vi "Visualizacion_NEW.vi"() -> ()   [LabVIEW 2021]
uses:
  <vilib>/Modbus/master/Modbus Master.lvclass
  4cb8985d-a683-42ab-be0b-9e8f42a2c2d0.vi
  <vilib>/Analysis/NI_AALBase.lvlib
  <vilib>/Modbus/master/Create Master Instance (TCP).vi
  <vilib>/Analysis/baseanly.llb/Mean (DBL).vi
panel:
  in  "Save Parameters":bool
  in  "Activar sim Bitron":bool
  out "MEDIA TEMPERATURAS":dbl format="%0.2f"
  out "Peltiers enable":bool
  out "Program Status":bool
  out "SP (T)":sgl
  out "Segmento_temp":u16
  in  "?":T1(tab)
  out "Temp Valve 1":sgl format="%#.2g"
  out "Temp Bobina 1":sgl
  out "PWM 1(SP)":u16
  out "PWM 2(SP)":u16
  out "Temp Valve 2":sgl format="%#.2g"
  out "Temp Bobina 2":sgl
  out "PWM 3(SP)":u16
  out "Temp Bobina 3":sgl
  out "Temp Valve 3":sgl format="%#.2g"
  out "PWM 4(SP)":u16
  out "Temp Valve 4":sgl format="%#.2g"
  out "Temp Bobina 4":sgl
  out "Temp Valve 5":sgl
  out "Temp Bobina 5":sgl
  out "PWM 5(SP)":u16
  out "PWM 6(SP)":u16
  out "Temp Valve 6":sgl format="%#.2g"
  out "Temp Bobina 6":sgl
  out "PWM 7(SP)":u16
  out "Temp Valve 7":sgl format="%#.2g"
  out "Temp Bobina 7":sgl
  out "PWM 8":u16
  out "Temp Bobina 8":sgl
  out "Temp Valve 8":sgl format="%#.2g"
  in  "?":T2(tab)
  in  "?":T3(tab)
  out "TEMPERATURA MEDIA":dynamicdata(graph)
  out "ALL TOGETHER":dynamicdata(graph)
  out "VALVULA 1 Y BOBINA 1":dynamicdata(graph)
  out "VALVULA 2 Y BOBINA 2":dynamicdata(graph)
  out "VALVULA 3 Y BOBINA 3":dynamicdata(graph)
  out "VALVULA 4 Y BOBINA 4":dynamicdata(graph)
  out "VALVULA 5  Y BOBINA 5":dynamicdata(graph)
  out "VALVULA 6 Y BOBINA 6":dynamicdata(graph)
  out "VALVULA 7 Y BOBINA 7":dynamicdata(graph)
  out "VALVULA 8 Y PELTIER 8":dynamicdata(graph)
  out "Camara climatica":dynamicdata(graph)
  out "W1.16":bool
  out "W1.15":bool
  out "W1.11":bool
  out "1.10":bool
  out "W1.14":bool
  out "W1.13":bool
  out "W1.12":bool
  out "W1.1":bool
  out "W2":bool
  out "W3":bool
  out "W4":bool
  out "W1.2":bool
  out "W1.3":bool
  out "W1.6":bool
  out "W1.5":bool
  out "W1.4":bool
  out "W1.9":bool
  out "W1.8":bool
  out "W1.7":bool
  out "warnings table":T4(array[cluster]) {"Time Stamp" format="%<%.3X %x>T"}
  in  "Reset":bool
  in  "Pelt ºC/min":dbl=2.5
  in  "Cam ºC/min":dbl=2.2
  in  "Tiempo máximo de ciclo(min)":dbl=90.0
  in  "Setpoint corte frío(ºC)":dbl=-30.0
  in  "Setpoint Frío(ºC)":dbl=-40.0
  in  "Setpoint peltiers(ºC)":dbl=85.0
  in  "Tiempo estabilidad de Frío(min)":dbl=15.0
  in  "Tiempo mínimo de ciclo(min)":dbl=70.0
  in  "Setpoint calor corte rampa(ºC)":dbl=51.0
  in  "T ciclo (Bitron FSM Sim)":dbl=90.0
  in  "Setpoint calor cam":dbl=55.0
  out "DO H2 Lab":bool
  in  "Guardar datos":bool=TRUE
  out "Array":dbl[][](array[numeric])
  out "Guardando en disco":bool
  out "array w/ subset deleted":dbl[][](array[numeric])
  out "Guardar Array":dbl[][](array[numeric])
  out "size(s)":i32
  out "senal_bitron":bool
  in  "Stop Control Program":bool
  out "Coils write":bool[](array[boolean])
  out "error out":errorcluster
  out "Int values":u16[](array[numeric])
  out "SGL values":sgl[](array[numeric])
  out "coil values":bool[](array[boolean])
  out "ComunicacionCRIO":bool
  out "current time":timestamp
  in  "run_program":bool
  out "Setpoint_temp_write":dbl
  out "Setpoint_hum_write":dbl
  out "Setpoint_temp_read":dbl
  out "Setpoint_hum_read":dbl
  in  "Pause_Entrar_camara":bool
  in  "Pause":bool
  in  "stop":bool
  # "Control Programa Principal"
  # "Cámara climática"
  # "ºC"
  # "ºC"
  # "%"
  # "%"
  # "Simulación señal Bitron"
  # "ºC"
  # "Peltier 1"
  # "ºC"
  # "ºC"
  # "Peltier 2"
  # "ºC"
  # "ºC"
  # "Peltier 3"
  # "ºC"
  # "ºC"
  # "Peltier 4"
  # "ºC"
  # "Peltier 5 (Doble)"
  # "ºC"
  # "ºC"
  # "Peltier 6 (Doble)"
  # "ºC"
  # "ºC"
  # "Peltier 7 (Doble)"
  # "ºC"
  # "ºC"
  # "Peltier 8 (Doble)"
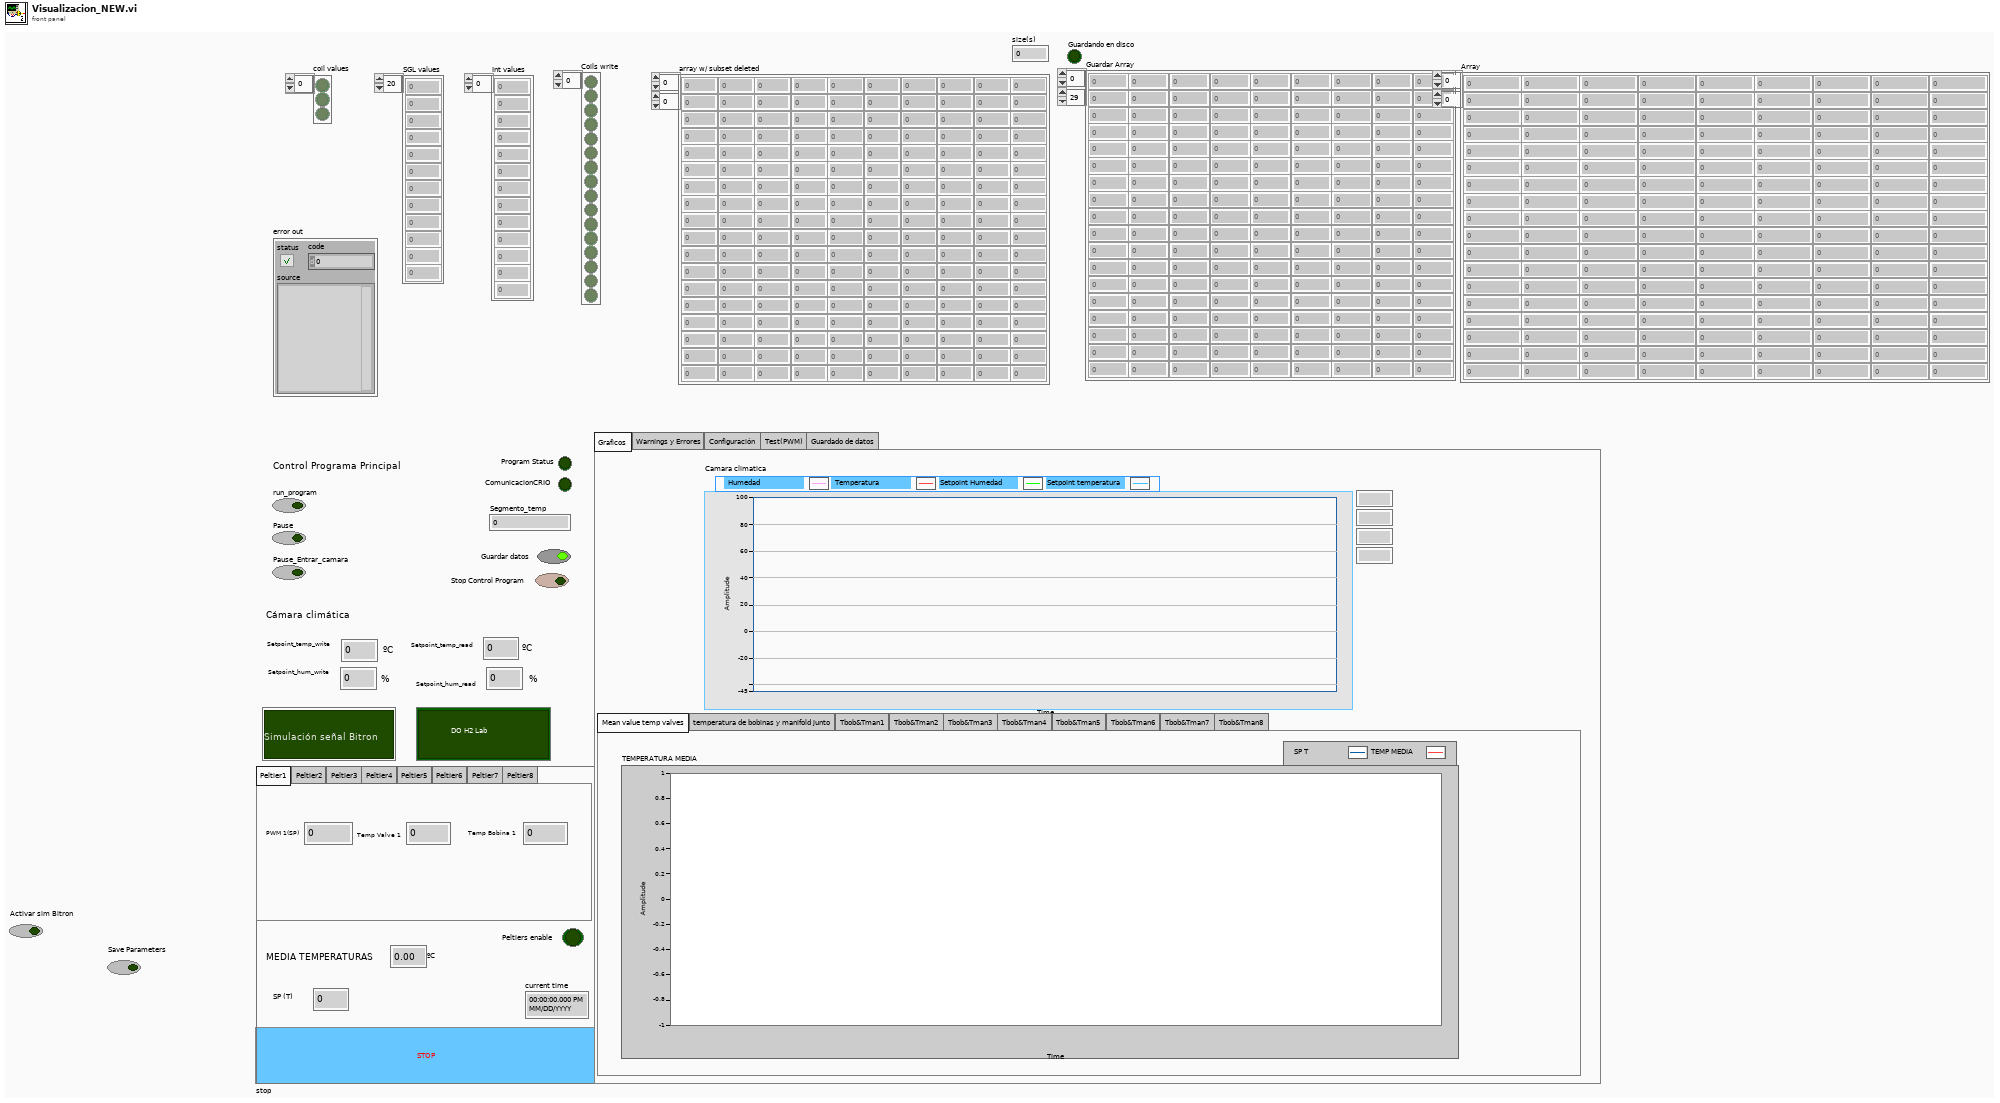
[diagram p1: front panel]
types:
  T1 = enum32{"Peltier1", "Peltier2", "Peltier3", "Peltier4", "Peltier5", "Peltier6", "Peltier7", "Peltier8"}
  T2 = enum32{"Graficos", "Warnings y Errores", "Configuración", "Test(PWM)", "Guardado de datos"}
  T3 = enum32{"Mean value temp valves", "temperatura de bobinas y manifold junto", "Tbob&Tman1", "Tbob&Tman2", "Tbob&Tman3", "Tbob&Tman4", "Tbob&Tman5", "Tbob&Tman6", "Tbob&Tman7", "Tbob&Tman8"}
  T4 = cluster{"Time Stamp":timestamp, "Descripcion":string, "Numeric":i32}[]
  T5 = enum16{"open", "open or create", "create or replace", "create", "open (read-only)"}
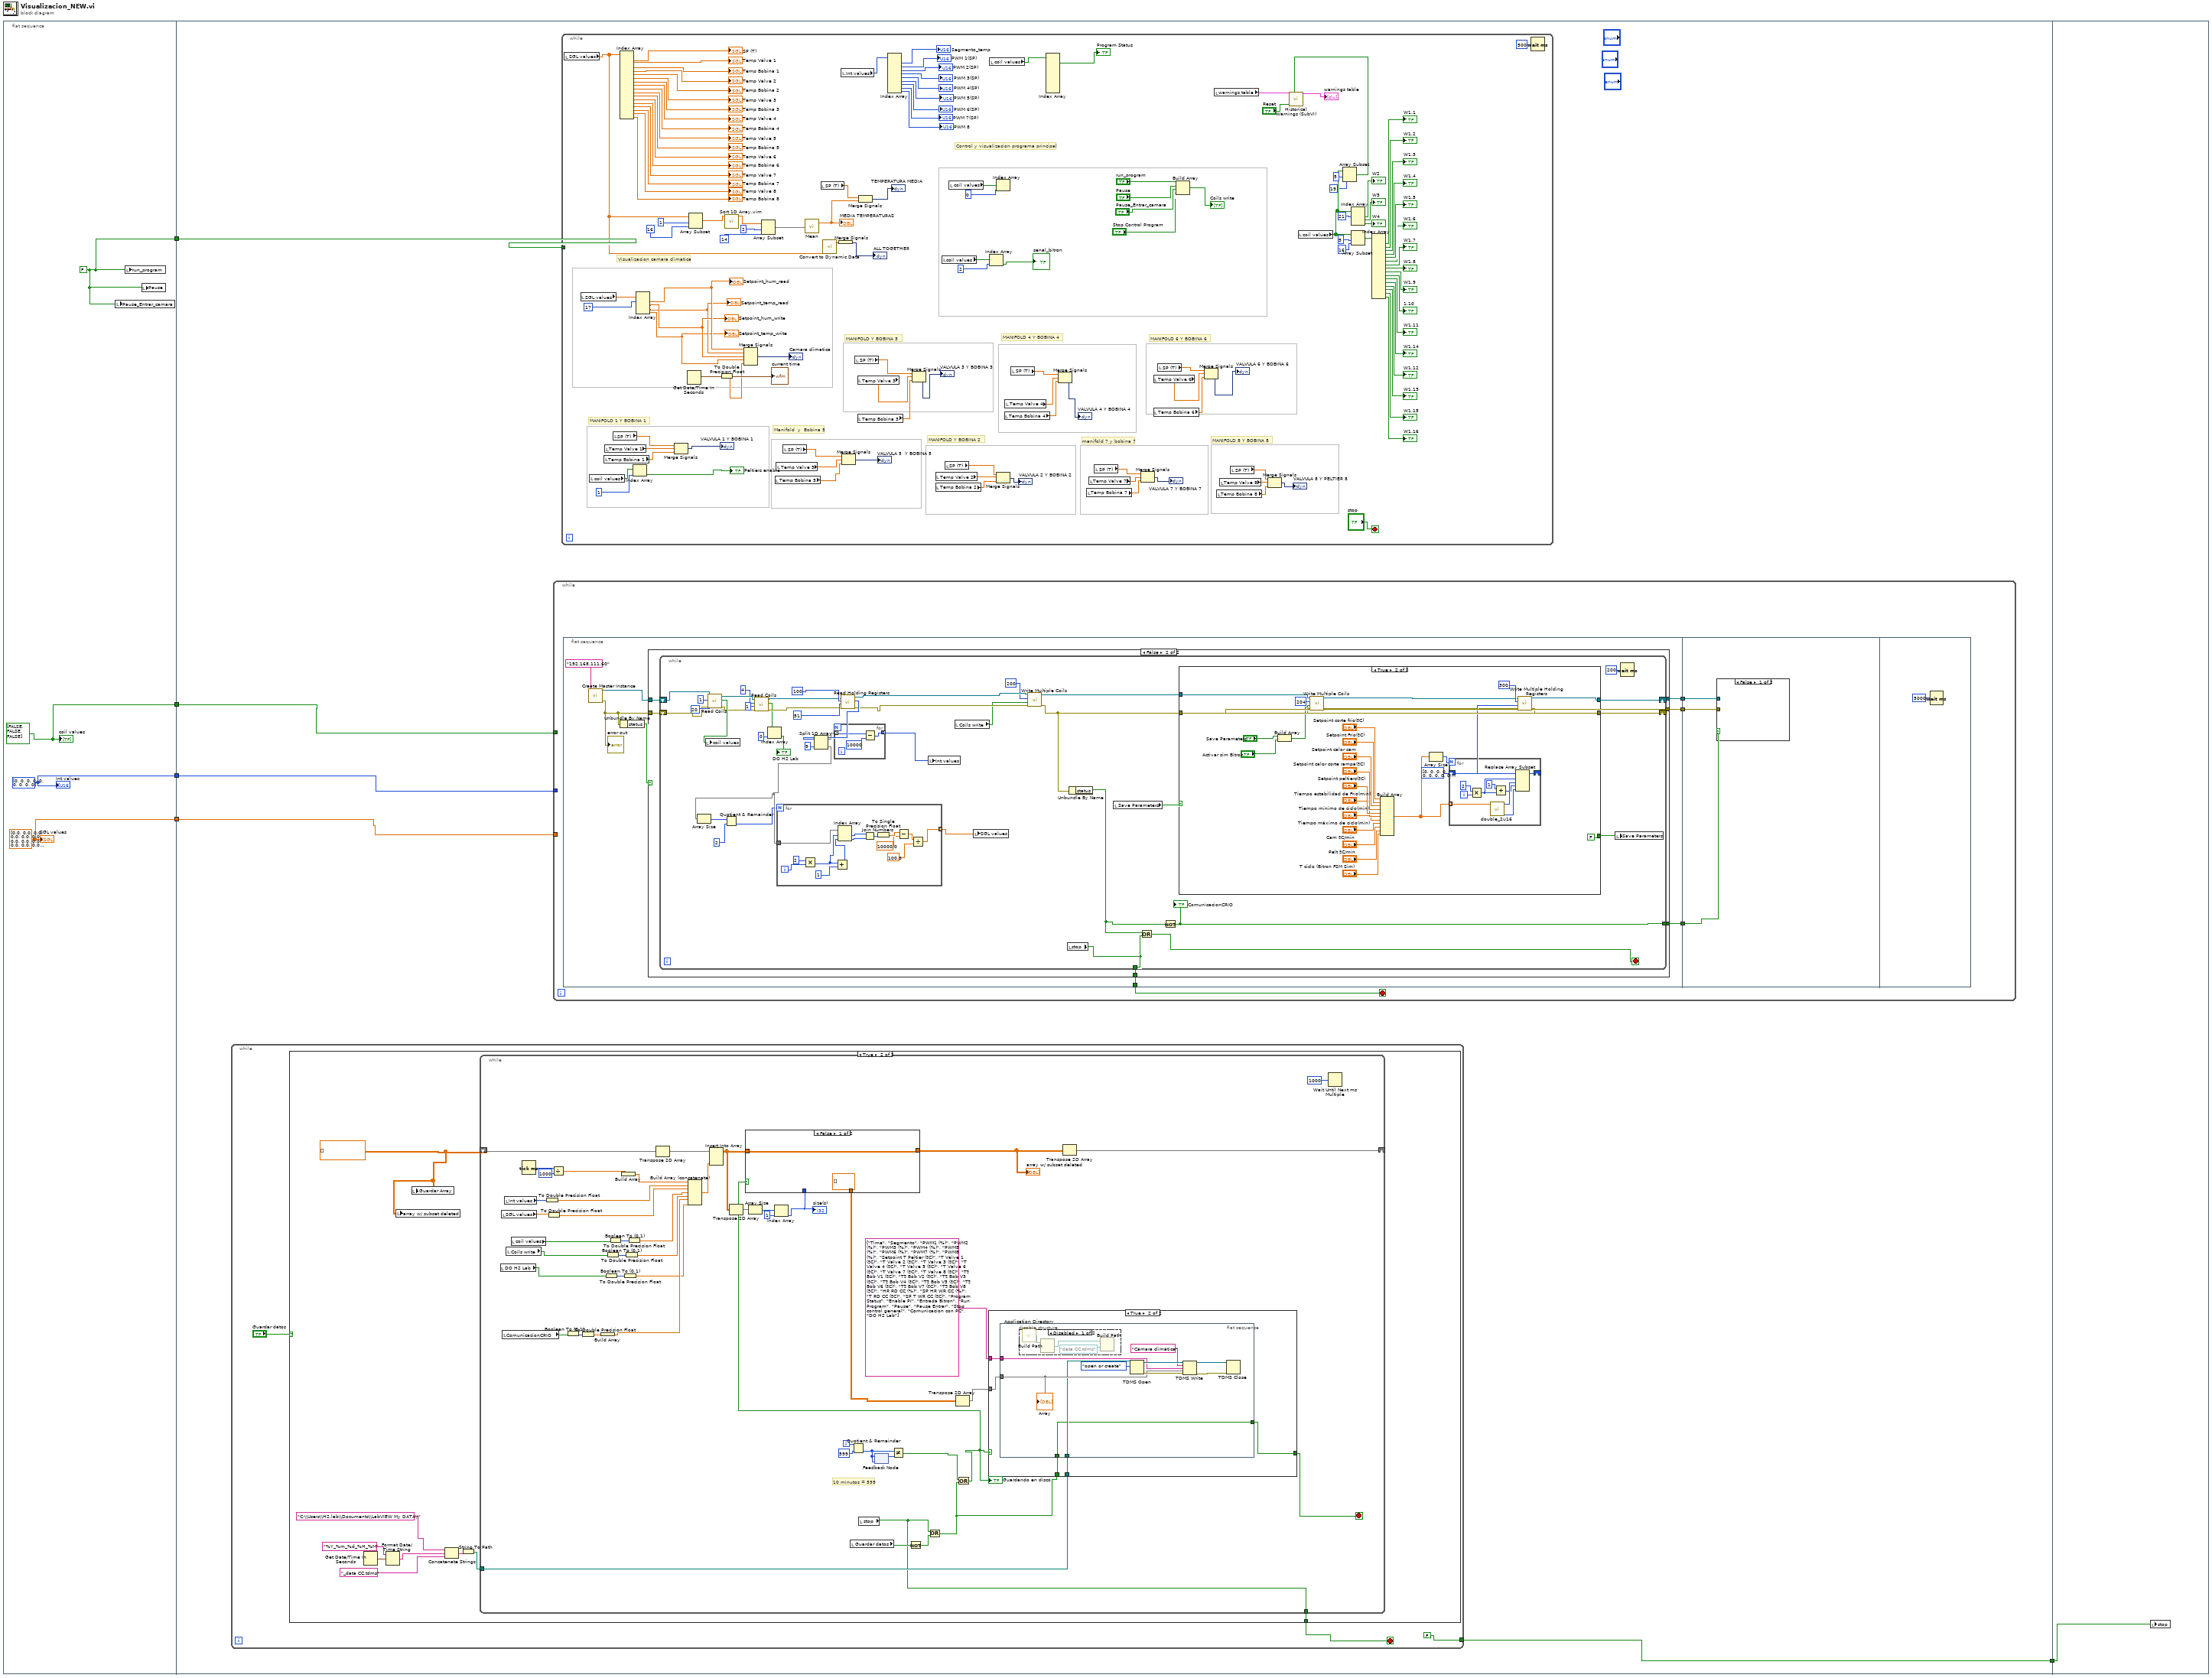
[diagram p0: block diagram]
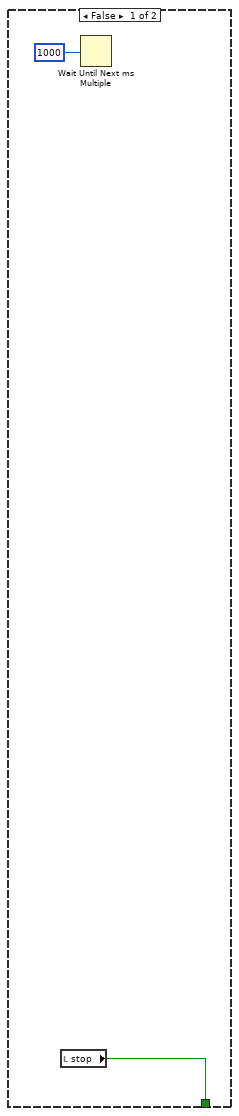
[diagram p2: hidden frame]
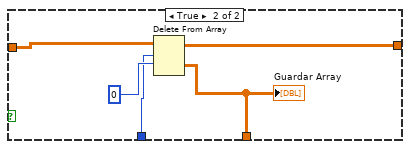
[diagram p3: hidden frame]
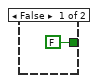
[diagram p4: hidden frame]
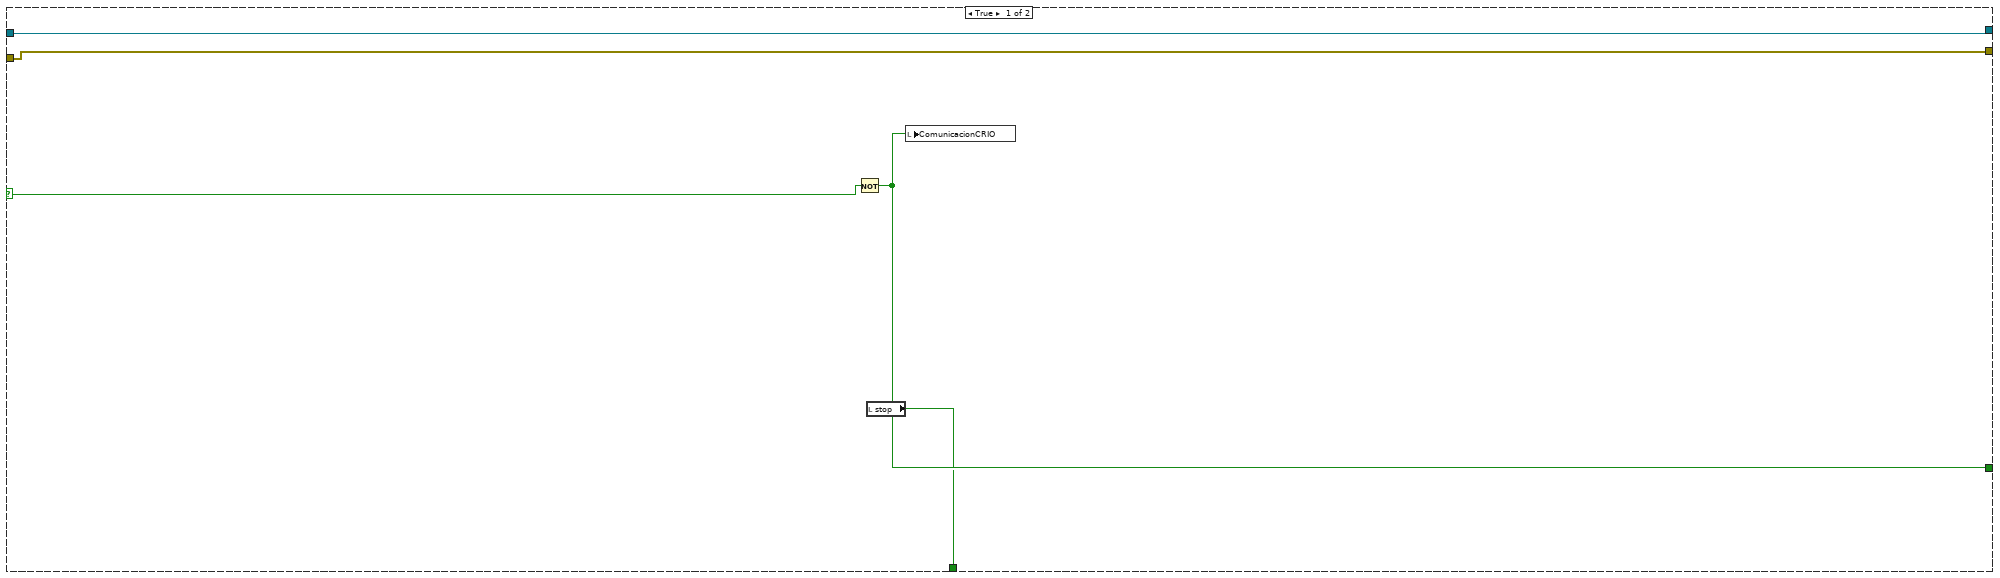
[diagram p6: hidden frame]
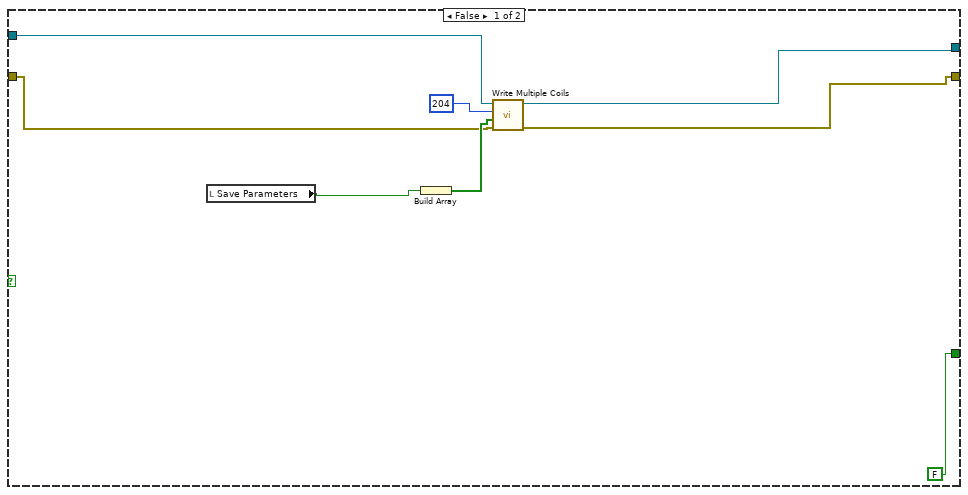
[diagram p7: hidden frame]
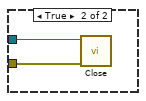
[diagram p8: hidden frame]
diagram:
  n1 = flat-sequence {
    tunnel: [w9] -> w5
    tunnel: [w8] -> w4
    tunnel: [w7] -> w3
    tunnel: [w6] -> w2
    tunnel: w5 -> [w14]
    tunnel: w4 -> [w13]
    tunnel: w3 -> [w12]
    tunnel: w2 -> [w11]
    tunnel: [w10] -> w1
    tunnel: w1 -> [w361]
    frame #0 {
      w7 = sgl[] [0.0, 0.0, 0.0, 0.0, 0.0, 0.0, 0.0, 0.0, 0.0, 0.0, 0.0, 0.0, 0.0, 0.0, 0.0, 0.0, 0.0, 0.0, 0.0, 0.0, 0.0] ("SGL values")
      w8 = u16[] [0, 0, 0, 0, 0, 0, 0, 0, 0] ("Int values")
      w6 = FALSE ("run_program")
      w9 = bool[] [FALSE, FALSE, FALSE] ("coil values")
      n2 = local write "Pause_Entrar_camara"(w6) -> ()
      n3 = local write "run_program"(w6) -> ()
      n4 = local write "Pause"(w6) -> ()
      "coil values" <- w9
      "Int values" <- w8
      "SGL values" <- w7
    }
    frame #1 {
      n5 = while {
        tunnel: [FALSE ("stop Control General")] -> w10
        stop <- w16 stop-if-true
        n6 = case shown="True" "Guardar datos" {
          tunnel: [w18 w20] -> w16
          frame False {
            n7 = local read "stop"() -> (w18:bool)
            n8 = Wait Until Next ms Multiple(millisecond multiple=u32 1000 ("milliseconds to wait")) -> ()  [unwired: 1 out]
          }
          frame True {
            w28 = dbl[][] []
            n9 = Get Date/Time In Seconds() -> (seconds since 1Jan1904=w27:timestamp)
            n10 = Format Date/Time String(time format string (%c)="%Y_%m_%d_%H_%M", seconds (now)=w27) -> (date/time string=w24:string)  [unwired: 1 in]
            n11 = local write "array w/ subset deleted"(w28) -> ()
            n12 = local write "Guardar Array"(w28) -> ()
            n13 = Concatenate Strings("C:\\Users\\H2.lab\\Documents\\LabVIEW My DATA\\" ("string"), w24, "_data CC.tdms" ("string")) -> (w25:string)
            n14 = String To Path(string=w25) -> (path=w22:path)
            n15 = while {
              shift-right: [w65] -> _
              shift-left: w28 -> [w68]
              tunnel: w22 -> [w56]
              tunnel: [w32] -> w20
              i -> [w73]
              stop <- w36 stop-if-true
              # "10 minutos = 599"
              n16 = local read "DO H2 Lab"() -> (w30:bool)
              n17 = local read "SGL values"() -> (w54:sgl[])
              n18 = local read "ComunicacionCRIO"() -> (w38:bool)
              n19 = local read "Int values"() -> (w55:u16[])
              n20 = local read "Coils write"() -> (w40:bool[])
              n21 = local read "coil values"() -> (w43:bool[])
              n22 = Tick Count (ms)() -> (millisecond timer value=w59:u32)
              n23 = To Double Precision Float(number=w55) -> (double precision float=w53:dbl[])
              n24 = To Double Precision Float(number=w54) -> (double precision float=w52:dbl[])
              n25 = Divide(x=w59, y=u32 1000) -> (x/y=w51:dbl)
              n26 = Boolean To (0,1)(Boolean=w38) -> (0, 1=w47:i16)
              n27 = To Double Precision Float(number=w47) -> (double precision float=w46:dbl)
              n28 = Build Array(w46) -> (w42:dbl[])
              n29 = Boolean To (0,1)(Boolean=w30) -> (0, 1=w31:i16)
              n30 = Boolean To (0,1)(Boolean=w40) -> (0, 1=w41:i16[])
              n31 = Boolean To (0,1)(Boolean=w43) -> (0, 1=w49:i16[])
              n32 = Build Array(w51) -> (w50:dbl[])
              n33 = To Double Precision Float(number=w31) -> (double precision float=w29:dbl)
              n34 = To Double Precision Float(number=w41) -> (double precision float=w39:dbl[])
              n35 = To Double Precision Float(number=w49) -> (double precision float=w48:dbl[])
              n36 = Transpose 2D Array(2D array=w68) -> (transposed array=w67:dbl[][])
              n37 = Build Array (concatenate)(w50, w53, w52, w48, w39, w42, w29) -> (w74:dbl[])
              n38 = Insert Into Array(array=w67, new element=w74) -> (w70:dbl[][])  [unwired: 2 in]
              n39 = Transpose 2D Array(2D array=w70) -> (transposed array=w64:dbl[][])
              n40 = Array Size(array=w64) -> (size(s)=w63:i32[])
              n41 = Index Array(array=w63, index=1) -> (element=w62:i32)
              "size(s)" <- w62
              n42 = local read "Guardar datos"() -> (w35:bool)
              n43 = Quotient & Remainder(x=w73, y=599) -> (floor(x/y)=w69:i32)  [unwired: 1 out]
              n44 = local read "stop"() -> (w32:bool)
              n45 = feedback-in #1(w69) -> ()
              n46 = feedback #1(w69) -> (w71:i32)
              n47 = Not Equal?(x=w69, y=w71) -> (x != y?=w37:bool)
              n48 = Not(x=w35) -> (.not. x?=w34:bool)
              n49 = Or(x=w32, y=w34) -> (x .or. y?=w33:bool)
              n50 = Or(x=w37, y=w33) -> (x .or. y?=w45:bool)
              "Guardando en disco" <- w45
              n51 = case shown="False" w45 {
                tunnel: w70 -> [w77 w80]
                tunnel: [w77 w82] -> w66
                tunnel: w62 -> [_ w79]
                tunnel: [dbl[][] [] w78] -> w44
                frame False {
                }
                frame True {
                  n52 = Delete From Array(array=w80, length=w79, index (row)=0) -> (deleted portion=w78:dbl[][], array with subset deleted=w82:dbl[][])  [unwired: 1 in]
                  "Guardar Array" <- w78
                }
              }
              "array w/ subset deleted" <- w66
              n53 = Transpose 2D Array(2D array=w44) -> (transposed array=w60:dbl[][])
              n54 = case shown="True" w45 {
                tunnel: string[] ["Time", "Segmento", "PWM1 (%)", "PWM2 (%)", "PWM3 (%)", "PWM4 (%)", "PWM5 (%)", "PWM6 (%)", "PWM7 (%)", "PWM8 (%)", "Setpoint T Peltier (ºC)", "T Valve 1 (ºC)", "T Valve 2 (ºC)", "T Valve 3 (ºC)", "T Valve 4 (ºC)", "T Valve 5 (ºC)", "T Valve 6 (ºC)", "T Valve 7 (ºC)", "T Valve 8 (ºC)", "Tª Bob V1 (ºC)", "Tª Bob V2 (ºC)", "Tª Bob V3 (ºC)", "Tª Bob V4 (ºC)", "Tª Bob V5 (ºC)", "Tª Bob V6 (ºC)", "Tª Bob V7 (ºC)", "Tª Bob V8 (ºC)", "HR RD CC (%)", "SP HR WR CC (%)", "T RD CC (ºC)", "SP T WR CC (ºC)", "Program Status", "Enable PI", "Entrada Bitron", "Run Program", "Pause", "Pause Entrar", "Stop control general", "Comunicacion con PC", "DO H2 Lab"] -> [_ w88]
                tunnel: w60 -> [_ w87]
                tunnel: w56 -> [_ w86]
                tunnel: w33 -> [_ w85]
                tunnel: [FALSE ("STOP ALL") w84] -> w36
                frame False {
                }
                frame True {
                  n55 = flat-sequence {
                    tunnel: w88 -> [w94]
                    tunnel: w87 -> [w91]
                    tunnel: w86 -> [w90]
                    tunnel: w85 -> [w89]
                    tunnel: [w89] -> w84
                    frame #0 {
                      n56 = disable-structure shown="Disabled" {
                        frame Disabled {
                          n57 = call <vilib>:"Application Directory.vi"() -> ("Application Directory"=w100:path)
                          n58 = Build Path(base path=w100) -> (appended path=w99:path)  [unwired: 1 in]
                          n59 = Build Path(base path=w99, name or relative path=path "data CC.tdms") -> ()  [unwired: 1 out]
                        }
                        frame Enabled {
                        }
                      }
                      n60 = TDMS Open(10:T5."open or create" ("operation (0:open)"), 11:w90) -> (0:w96:errorcluster, 3:w97:refnum<k34>)  [unwired: 5 in]
                      n61 = TDMS Write(0:w97, 5:"Cámara climática" ("group name in (Untitled)"), 7:w94, 9:w91, 11:w96) -> (4:w93:refnum<k34>, 15:w92:errorcluster)  [unwired: 1 in, 2 out]
                      n62 = TDMS Close(8:w92, 11:w93) -> ()  [unwired: 2 out]
                      "Array" <- w91
                    }
                  }
                }
              }
              n63 = Transpose 2D Array(2D array=w66) -> (transposed array=w65:dbl[][])
              n64 = Wait Until Next ms Multiple(millisecond multiple=u32 1000 ("milliseconds to wait")) -> ()  [unwired: 1 out]
            }
          }
        }
      }
      n65 = while {
        tunnel: w14 -> [_]
        tunnel: w13 -> [_]
        tunnel: w12 -> [_]
        stop <- w102 stop-if-true
        n66 = flat-sequence {
          tunnel: [w111] -> w105
          tunnel: [w110] -> w104
          tunnel: [w109] -> w103
          tunnel: [w108] -> w102
          tunnel: w105 -> [w229]
          tunnel: w104 -> [w228]
          tunnel: w103 -> [w227]
          frame #0 {
            n67 = call-poly <vilib>:"Create Master Instance.vi"("address"="192.168.111.60") -> ("error out"=w107:errorcluster, "TCP master instance"=w112:refnum<class "Modbus Master.lvclass">)  [unwired: 9 in]
            "error out" <- w107
            n68 = Unbundle By Name(w107) -> ("status"=w106:bool)
            n69 = case shown="False" w106 {
              selector: w106 -> [w115 _]
              tunnel: w112 -> [w118 w124]
              tunnel: [w116 w123] -> w111
              tunnel: [w118 w122] -> w110
              tunnel: [w117 w121] -> w109
              tunnel: [w114 w120] -> w108
              tunnel: w107 -> [w117 w119]
              frame True {
                n70 = Not(x=w115) -> (.not. x?=w116:bool)
                n71 = local read "stop"() -> (w114:bool)
                n72 = local write "ComunicacionCRIO"(w116) -> ()
              }
              frame False {
                n73 = while {
                  shift-right: [w126] -> w122
                  shift-left: w124 -> [w153]
                  shift-right: [w125] -> w121
                  shift-left: w119 -> [w152]
                  tunnel: [w149] -> w123
                  tunnel: [w147] -> w120
                  stop <- w151 stop-if-true
                  n74 = call-dynamic "Read Coils.vi"("error in (no error)"=w152, "number of coils"=u16 20, "starting address"=u16 1, "Modbus master in"=w153) -> ("error out"=w138:errorcluster, "coil values"=w142:bool[], "Modbus master out"=w139:refnum<class "Modbus Master.lvclass">)  [unwired: 5 in]
                  n75 = local write "coil values"(w142) -> ()
                  n76 = call-dynamic "Read Coils.vi"("error in (no error)"=w138, "number of coils"=u16 1, "starting address"=u16 4, "Modbus master in"=w139) -> ("error out"=w136:errorcluster, "coil values"=w133:bool[], "Modbus master out"=w137:refnum<class "Modbus Master.lvclass">)  [unwired: 5 in]
                  n77 = Index Array(array=w133, index=0) -> (element=→"DO H2 Lab":bool)
                  n78 = call-dynamic "Read Holding Registers.vi"("error in (no error)"=w136, "number of holding registers"=u16 51, "starting address"=u16 100, "Modbus master in"=w137) -> ("error out"=w145:errorcluster, "register values"=w155:u16[], "Modbus master out"=w146:refnum<class "Modbus Master.lvclass">)  [unwired: 5 in]
                  n79 = Split 1D Array(array=w155, index=9) -> (first subarray=w154:u16[], second subarray=w159:u16[])
                  n80 = Array Size(array=w159) -> (size(s)=w158:i32)
                  n81 = Quotient & Remainder(x=w158, y=2) -> (floor(x/y)=w156:i32)  [unwired: 1 out]
                  n82 = for {
                    N: w156 -> [_]
                    tunnel: w159 -> [w219]
                    tunnel: [w216] -> w140 mode=indexing
                    i -> [w226]
                    n83 = Multiply(x=2, y=w226) -> (x*y=w224:i32)
                    n84 = Add(x=w224, y=1) -> (x+y=w222:i32)
                    n85 = Index Array(array=w219, index #1=w224, index #2=w222) -> (element #1=w221:u16, element #2=w220:u16)
                    n86 = Join Numbers(hi=w221, lo=w220) -> ((hi.lo)=w218:u32)
                    n87 = To Single Precision Float(number=w218) -> (single precision float=w215:sgl)
                    n88 = Subtract(x=w215, y=sgl 10000.0) -> (x-y=w213:sgl)
                    n89 = Divide(x=w213, y=sgl 100.0) -> (x/y=w216:sgl)
                  }
                  n90 = for {
                    tunnel: w154 -> [w212] mode=indexing
                    tunnel: [w210] -> w141 mode=indexing
                    n91 = Subtract(x=w212, y=u16 10000) -> (x-y=w210:u16)
                  }
                  n92 = local write "Int values"(w141) -> ()
                  n93 = local read "Coils write"() -> (w143:bool[])
                  n94 = local write "SGL values"(w140) -> ()
                  n95 = call-dynamic "Write Multiple Coils.vi"("error in (no error)"=w145, "coil values"=w143, "starting address"=u16 200, "Modbus master in"=w146) -> ("error out"=w127:errorcluster, "Modbus master out"=w128:refnum<class "Modbus Master.lvclass">)  [unwired: 6 in]
                  n96 = local read "stop"() -> (w147:bool)
                  n97 = Unbundle By Name(w127) -> ("status"=w150:bool)
                  n98 = local read "Save Parameters"() -> (w130:bool)
                  n99 = Or(x=w150, y=w147) -> (x .or. y?=w151:bool)
                  n100 = Not(x=w150) -> (.not. x?=w149:bool)
                  "ComunicacionCRIO" <- w149
                  n101 = case shown="True" w130 {
                    tunnel: [FALSE ("Save Parameters") FALSE ("Save Parameters")] -> w129
                    tunnel: w128 -> [w168 w176]
                    tunnel: w127 -> [w167 w175]
                    tunnel: [w166 w174] -> w126
                    tunnel: [w165 w173] -> w125
                    frame False {
                      n102 = local read "Save Parameters"() -> (w169:bool)
                      n103 = Build Array(w169) -> (w171:bool[])
                      n104 = call-dynamic "Write Multiple Coils.vi"("error in (no error)"=w167, "coil values"=w171, "starting address"=u16 204, "Modbus master in"=w168) -> ("error out"=w165:errorcluster, "Modbus master out"=w166:refnum<class "Modbus Master.lvclass">)  [unwired: 6 in]
                    }
                    frame True {
                      n105 = Build Array("Save Parameters", "Activar sim Bitron") -> (w180:bool[])
                      n106 = call-dynamic "Write Multiple Coils.vi"("error in (no error)"=w175, "coil values"=w180, "starting address"=u16 204, "Modbus master in"=w176) -> ("error out"=w179:errorcluster, "Modbus master out"=w178:refnum<class "Modbus Master.lvclass">)  [unwired: 6 in]
                      n107 = Build Array("Setpoint corte frío(ºC)", "Setpoint Frío(ºC)", "Setpoint calor cam", "Setpoint calor corte rampa(ºC)", "Setpoint peltiers(ºC)", "Tiempo estabilidad de Frío(min)", "Tiempo mínimo de ciclo(min)", "Tiempo máximo de ciclo(min)", "Cam ºC/min", "Pelt ºC/min", "T ciclo (Bitron FSM Sim)") -> (w187:dbl[])
                      n108 = Array Size(array=w187) -> (size(s)=w186:i32)
                      n109 = for {
                        N: w186 -> [_]
                        shift-right: [w201] -> w184
                        shift-left: u16[] [0, 0, 0, 0, 0, 0, 0, 0, 0, 0, 0, 0, 0, 0, 0, 0, 0, 0, 0, 0, 0, 0] -> [w202]
                        tunnel: w187 -> [w200] mode=indexing
                        i -> [w209]
                        n110 = Multiply(x=2, y=w209) -> (x*y=w205:i32)
                        n111 = call "double_2u16.vi"("Entrada"=w200) -> ("Salida 2"=w206:u16, "Salida 1"=w207:u16)  [unwired: 9 in]
                        n112 = Add(x=1, y=w205) -> (x+y=w203:i32)
                        n113 = Replace Array Subset(array=w202, new element #1=w207, index #1=w205, new element #2=w206, index #2=w203) -> (w201:u16[])
                      }
                      n114 = call-dynamic "Write Multiple Holding Registers.vi"("error in (no error)"=w179, "holding register values"=w184, "starting address"=u16 300, "Modbus master in"=w178) -> ("error out"=w173:errorcluster, "Modbus master out"=w174:refnum<class "Modbus Master.lvclass">)  [unwired: 6 in]
                    }
                  }
                  n115 = local write "Save Parameters"(w129) -> ()
                  n116 = Wait (ms)(milliseconds to wait=u32 200) -> ()  [unwired: 1 out]
                }
              }
            }
          }
          frame #1 {
            n117 = case shown="False" w229 {
              tunnel: w228 -> [_ w231]
              tunnel: w227 -> [_ w230]
              frame False {
              }
              frame True {
                n118 = call-dynamic "Close.vi"("error in (no error)"=w230, "Modbus master in"=w231) -> ()  [unwired: 9 in, 1 out]
              }
            }
          }
          frame #2 {
            n119 = Wait (ms)(milliseconds to wait=u32 5000) -> ()  [unwired: 1 out]
          }
        }
      }
      n120 = while {
        tunnel: w11 -> [_]
        stop <- "stop" stop-if-true
        # "MANIFOLD 8 Y BOBINA 8"
        # "manifold 7 y bobina 7"
        # "MANIFOLD 6 Y BOBINA 6"
        # "MANIFOLD 4 Y BOBINA 4"
        # "MANIFOLD Y BOBINA 3"
        # "MANIFOLD Y BOBINA 2"
        # "Manifold  y  Bobina 5"
        # "MANIFOLD 1 Y BOBINA 1"
        # "Visualizacion camara climatica"
        # "Control y visualizacion programa principal"
        n121 = local read "SGL values"() -> (w265:sgl[])
        n122 = local read "SGL values"() -> (w355:sgl[])
        n123 = local read "coil values"() -> (w349:bool[])
        n124 = local read "Temp Bobina 1"() -> (w328:sgl)
        n125 = local read "Temp Valve 1"() -> (w329:sgl)
        n126 = local read "SP (T)"() -> (w330:sgl)
        n127 = Index Array(array=w265) -> (element #1=→"SP (T)":sgl, element #2=→"Temp Valve 1":sgl, element #3=→"Temp Bobina 1":sgl, element #4=→"Temp Valve 2":sgl, element #5=→"Temp Bobina 2":sgl, element #6=→"Temp Valve 3":sgl, element #7=→"Temp Bobina 3":sgl, element #8=→"Temp Valve 4":sgl, element #9=→"Temp Bobina 4":sgl, element #10=→"Temp Valve 5":sgl, element #11=→"Temp Bobina 5":sgl, element #12=→"Temp Valve 6":sgl, element #13=→"Temp Bobina 6":sgl, element #14=→"Temp Valve 7":sgl, element #15=→"Temp Bobina 7":sgl, element #16=→"Temp Valve 8":sgl, element #17=→"Temp Bobina 8":sgl)  [unwired: 17 in]
        n128 = Index Array(array=w349, index=1) -> (element=→"Peltiers enable":bool)
        n129 = Index Array(array=w355, index #1=17 ("index")) -> (element #1=w353:sgl, element #2=w352:sgl, element #3=w351:sgl, element #4=w350:sgl)  [unwired: 3 in]
        "Setpoint_hum_read" <- w353
        "Setpoint_temp_read" <- w351
        "Setpoint_hum_write" <- w352
        "Setpoint_temp_write" <- w350
        n130 = Merge Signals(w330, w329, w328) -> (→"VALVULA 1 Y BOBINA 1":dynamicdata)
        n131 = Get Date/Time In Seconds() -> (seconds since 1Jan1904=w358:timestamp)
        "current time" <- w358
        n132 = Array Subset(array=w265, index=1, length=16) -> (w274:sgl[])
        n133 = To Double Precision Float(number=w358) -> (double precision float=w357:dbl)
        n134 = call "Sort 1D Array.vim"("unsorted array"=w274) -> ("sorted array"=w273:sgl[])  [unwired: 10 in]
        n135 = Merge Signals(w353, w351, w352, w350, w357) -> (→"Camara climatica":dynamicdata)
        n136 = Array Subset(array=w273, index=2, length=14) -> (w270:sgl[])
        n137 = local read "Temp Bobina 5"() -> (w301:sgl)
        n138 = local read "Temp Valve 5"() -> (w302:sgl)
        n139 = local read "SP (T)"() -> (w303:sgl)
        n140 = call-poly <vilib>:"Mean.vi"("X"=w270) -> ("mean"=w268:dbl)  [unwired: 1 out]
        "MEDIA TEMPERATURAS" <- w268
        n141 = local read "SP (T)"() -> (w269:sgl)
        n142 = call "Convert to Dynamic Data"("Array"=w265) -> ("Dynamic Data Type"=w264:dynamicdata)  [unwired: 3 in]
        n143 = Merge Signals(w264) -> (→"ALL TOGETHER":dynamicdata)
        n144 = local read "Int values"() -> (w315:u16[])
        n145 = Merge Signals(w303, w302, w301) -> (→"VALVULA 5  Y BOBINA 5":dynamicdata)
        n146 = local read "SP (T)"() -> (w297:sgl)
        n147 = local read "Temp Valve 3"() -> (w296:sgl)
        n148 = local read "Temp Bobina 3"() -> (w295:sgl)
        n149 = Merge Signals(w269, w268) -> (→"TEMPERATURA MEDIA":dynamicdata)
        n150 = Index Array(array=w315) -> (element #1=→"Segmento_temp":u16, element #2=→"PWM 1(SP)":u16, element #3=→"PWM 2(SP)":u16, element #4=→"PWM 3(SP)":u16, element #5=→"PWM 4(SP)":u16, element #6=→"PWM 5(SP)":u16, element #7=→"PWM 6(SP)":u16, element #8=→"PWM 7(SP)":u16, element #9=→"PWM 8":u16)  [unwired: 9 in]
        n151 = Merge Signals(w297, w296, w295) -> (→"VALVULA 3 Y BOBINA 3":dynamicdata)
        n152 = local read "Temp Valve 2"() -> (w290:sgl)
        n153 = local read "Temp Bobina 2"() -> (w289:sgl)
        n154 = local read "coil values"() -> (w339:bool[])
        n155 = local read "SP (T)"() -> (w299:sgl)
        n156 = local read "coil values"() -> (w346:bool[])
        n157 = Index Array(array=w339, index=2) -> (element=→"senal_bitron":bool)
        n158 = local read "coil values"() -> (w305:bool[])
        n159 = Index Array(array=w346, index=0) -> ()  [unwired: 1 out]
        n160 = Merge Signals(w299, w290, w289) -> (→"VALVULA 2 Y BOBINA 2":dynamicdata)
        n161 = local read "Temp Bobina 4"() -> (w291:sgl)
        n162 = local read "Temp Valve 4"() -> (w292:sgl)
        n163 = local read "SP (T)"() -> (w293:sgl)
        n164 = Index Array(array=w305) -> (element #1=→"Program Status":bool)  [unwired: 9 in, 8 out]
        n165 = Merge Signals(w293, w292, w291) -> (→"VALVULA 4 Y BOBINA 4":dynamicdata)
        n166 = local read "Temp Bobina 7"() -> (w282:sgl)
        n167 = local read "Temp Valve 7"() -> (w283:sgl)
        n168 = local read "SP (T)"() -> (w284:sgl)
        n169 = Merge Signals(w284, w283, w282) -> (→"VALVULA 7 Y BOBINA 7":dynamicdata)
        n170 = local read "Temp Valve 6"() -> (w287:sgl)
        n171 = local read "Temp Bobina 6"() -> (w288:sgl)
        n172 = local read "SP (T)"() -> (w286:sgl)
        n173 = Build Array("run_program", "Pause", "Pause_Entrar_camara", "Stop Control Program") -> (→"Coils write":bool[])
        n174 = Merge Signals(w286, w287, w288) -> (→"VALVULA 6 Y BOBINA 6":dynamicdata)
        n175 = local read "warnings table"() -> (w238:T4)
        n176 = local read "Temp Bobina 8"() -> (w277:sgl)
        n177 = local read "Temp Valve 8"() -> (w278:sgl)
        n178 = local read "SP (T)"() -> (w279:sgl)
        n179 = Merge Signals(w279, w278, w277) -> (→"VALVULA 8 Y PELTIER 8":dynamicdata)
        n180 = local read "coil values"() -> (w237:bool[])
        n181 = Array Subset(array=w237, index=5, length=19) -> (w234:bool[])
        n182 = call "Historical Warnings (SubVI).vi"("Warnings bool array"=w234, "in"="Reset", "warnings table in"=w238) -> ("Warnings table out"=→"warnings table":T4)  [unwired: 8 in]
        n183 = Index Array(array=w237, index #1=21 ("index")) -> (element #1=→"W2":bool, element #2=→"W3":bool, element #3=→"W4":bool)  [unwired: 2 in]
        n184 = Array Subset(array=w237, index=5, length=16) -> (w256:bool[])
        n185 = Index Array(array=w256) -> (element #1=→"W1.1":bool, element #2=→"W1.2":bool, element #3=→"W1.3":bool, element #4=→"W1.4":bool, element #5=→"W1.5":bool, element #6=→"W1.6":bool, element #7=→"W1.7":bool, element #8=→"W1.8":bool, element #9=→"W1.9":bool, element #10=→"1.10":bool, element #11=→"W1.11":bool, element #12=→"W1.14":bool, element #13=→"W1.12":bool, element #14=→"W1.13":bool, element #15=→"W1.15":bool, element #16=→"W1.16":bool)  [unwired: 16 in]
        n186 = Wait (ms)(milliseconds to wait=u32 500) -> ()  [unwired: 1 out]
      }
    }
    frame #2 {
      n187 = local write "stop"(w361) -> ()
    }
  }
